vi "sdf.vi"(3 "assets":string) -> (1 "sdf out":string)   [LabVIEW 2012]
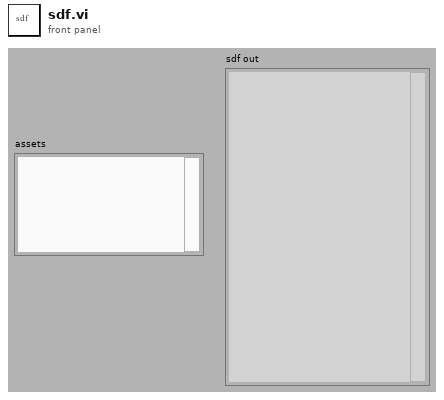
[diagram p1: front panel]
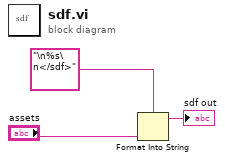
[diagram p0: block diagram]
diagram:
  n1 = Format Into String(format string="\n%s\n</sdf>", "assets") -> (resulting string=→"sdf out":string)  [unwired: 2 in, 1 out]
